vi "JSON to Map.vi"(6 "LVClass Serializer":refnum<class "JSONtext LVClass Serializer.lvclass">, 8 "error in (no error)":errorcluster, 9 "Map Type in":variant, 10 "Offset":i32, 11 "<JSON>":string) -> (0 "error out":errorcluster, 1 "Map":variant)   [LabVIEW 2020, in "JSONtext.lvlib" / "SetMap.lvlib"]
uses:
  <vilib>/JDP Science/JSONtext/support/Set Map/SetMap.lvlib
  <vilib>/JDP Science/JSONtext/LVClass Serializer/JSONtext LVClass Serializer.lvclass
  <vilib>/JDP Science/JSONtext/support/Set Map/SubType.vi
  <vilib>/Utility/Data Type/NI_Data Type.lvlib
  <vilib>/JDP Science/JSONtext/JSONtext.lvlib
  <vilib>/JDP Science/JDP Science Common Utilities/JDP Utility.lvlib
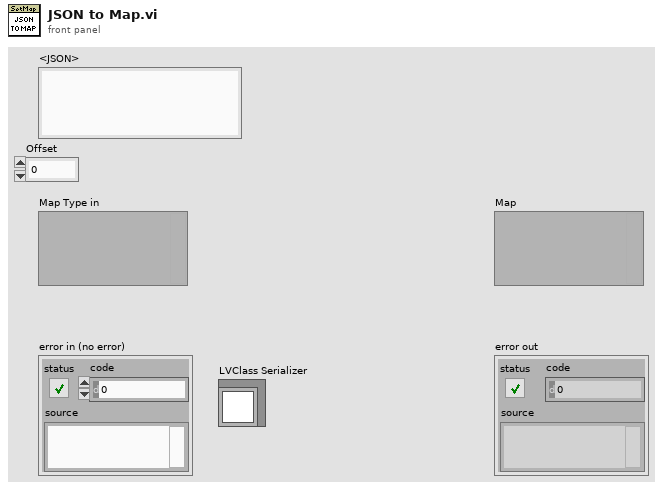
[diagram p1: front panel]
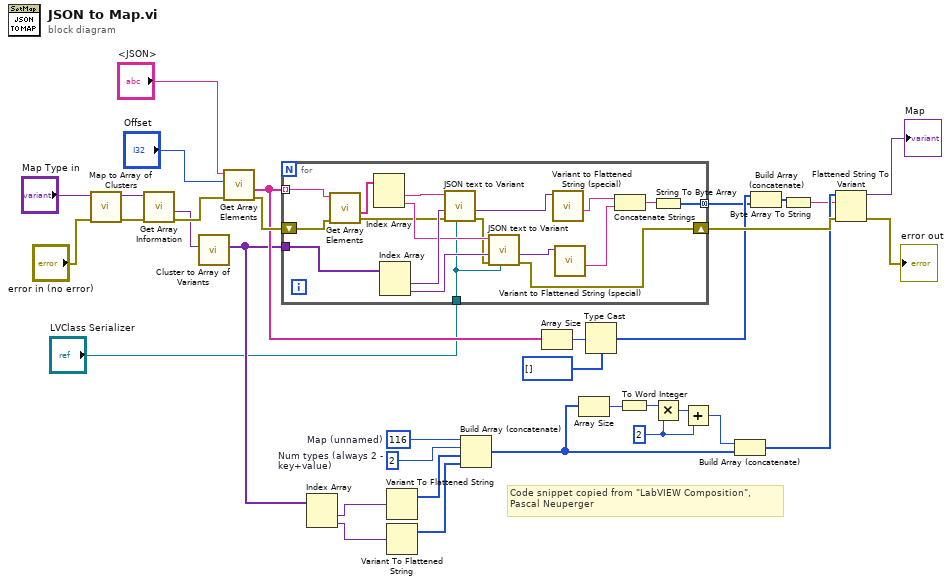
[diagram p0: block diagram]
diagram:
  w15 = i16 2 ("x")
  w9 = i16 2  # Num types (always 2 - key+value)
  w8 = i16 116  # Map (unnamed)
  # "Code snippet copied from \"LabVIEW Composition\",\nPascal Neuperger"
  n1 = call <vilib>:"Map to Array of Clusters.vi"("error in"="error in (no error)", "Map"="Map Type in") -> ("error out"=w29:errorcluster, "Array of Clusters (key-value)"=w3:variant)  [unwired: 8 in]
  n2 = call <vilib>:"Get Array Information.vi"("error in (no error)"=w29, "variant"=w3) -> ("error out"=w30:errorcluster, "array element data type"=w5:variant)  [unwired: 6 in, 2 out]
  n3 = call <vilib>:"Cluster to Array of Variants.vi"("Cluster"=w5) -> ("Array of Cluster Elements"=w16:variant[])  [unwired: 10 in]
  n4 = call <vilib>:"Get Array Elements.vi"("error in (no error)"=w30, "Offset"="Offset", "JSON"="<JSON>") -> ("error out"=w31:errorcluster, "<JSON>"=w25:string[])  [unwired: 6 in, 1 out]
  n5 = for {
    tunnel: w25 -> [w52] mode=indexing
    tunnel: w16 -> [w49]
    tunnel: [w42] -> w19 mode=concatenating
    shift-right: [w38] -> w32
    shift-left: w31 -> [w41]
    tunnel: "LVClass Serializer" -> [w37]
    n6 = call <vilib>:"Get Array Elements.vi"("error in (no error)"=w41, "JSON"=w52) -> ("error out"=w40:errorcluster, "<JSON>"=w51:string[])  [unwired: 7 in, 1 out]
    n7 = Index Array(array=w51) -> (element #1=w50:string, element #2=w47:string)  [unwired: 2 in]
    n8 = Index Array(array=w49) -> (element #1=w48:variant, element #2=w46:variant)  [unwired: 2 in]
    n9 = call <vilib>:"JSON text to Variant.vi"("LVClass Serializer"=w37, "error in (no error)"=w40, "Data Type"=w48, "JSON"=w50) -> ("error out"=w39:errorcluster, "Variant out"=w35:variant)  [unwired: 6 in]
    n10 = call <vilib>:"JSON text to Variant.vi"("LVClass Serializer"=w37, "error in (no error)"=w39, "Data Type"=w46, "JSON"=w47) -> ("error out"=w38:errorcluster, "Variant out"=w36:variant)  [unwired: 6 in]
    n11 = call <vilib>:"Variant to Flattened String (special).vi"("Variant"=w35) -> ("data"=w45:string)  [unwired: 9 in, 1 out]
    n12 = call <vilib>:"Variant to Flattened String (special).vi"("Variant"=w36) -> ("data"=w44:string)  [unwired: 9 in, 1 out]
    n13 = Concatenate Strings(w45, w44) -> (w43:string)
    n14 = String To Byte Array(string=w43) -> (unsigned byte array=w42:u8[])
  }
  n15 = Index Array(array=w16) -> (element #1=w17:variant, element #2=w18:variant)  [unwired: 2 in]
  n16 = Variant To Flattened String(Variant=w17) -> (1:w6:i16[])  [unwired: 1 out]
  n17 = Variant To Flattened String(Variant=w18) -> (1:w7:i16[])  [unwired: 1 out]
  n18 = Build Array (concatenate)(w8, w9, w6, w7) -> (w11:i16[])
  n19 = Array Size(array=w25) -> (size(s)=w23:i32)
  n20 = Array Size(array=w11) -> (size(s)=w10:i32)
  n21 = Type Cast(type=u8[] [], x=w23) -> (*(type *) &x=w27:u8[])
  n22 = To Word Integer(number=w10) -> (16bit integer=w12:i16)
  n23 = Multiply(x=w12, y=w15) -> (x*y=w13:i16)
  n24 = Add(x=w13, y=w15) -> (x+y=w14:i16)
  n25 = Build Array (concatenate)(w14, w11) -> (w21:i16[])
  n26 = Build Array (concatenate)(w27, w19) -> (w26:u8[])
  n27 = Byte Array To String(unsigned byte array=w26) -> (string=w20:string)
  n28 = Flattened String To Variant(4:w32, 6:w20, 7:w21) -> (0:→"error out":errorcluster, 3:→"Map":variant)
